vi "Decompose Map - Variant Mixed Value - Decomposes Successfully.vi"() -> ()   [LabVIEW 2019]
uses:
  <vilib>/addons/_JKI Toolkits/Caraya/classes/Assert/Assert Equal Value_Variant.vi
  Composition/Composition.lvlib
  <vilib>/addons/_JKI Toolkits/Caraya/classes/Test/Test.lvclass
  <vilib>/addons/_JKI Toolkits/Caraya/classes/Assert/Assert.lvclass
panel:
  out "error out":errorcluster
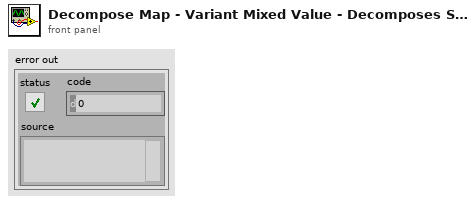
[diagram p1: front panel]
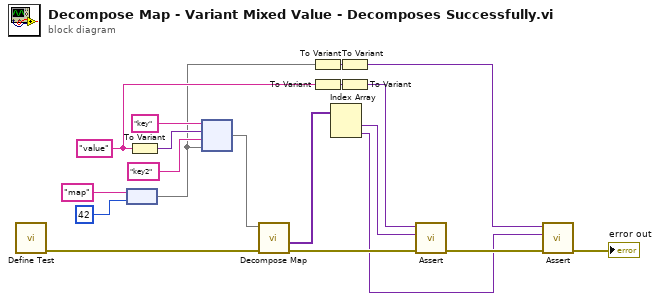
[diagram p0: block diagram]
diagram:
  w16 = "value" ("key")
  n1 = call <vilib>:"Define Test.vi"() -> ("error out"=w15:errorcluster)  [unwired: 10 in, 1 out]
  n2 = node("map" ("key"), 42 ("value")) -> (w2:map{string, i32})
  n3 = To Variant(anything=w16) -> (Variant=w14:variant)
  n4 = node("key" ("key"), w14, "key2" ("key"), w2) -> (w13:map{string, variant})
  n5 = call "Decompose Map.vi"("error in (no error)"=w15, "Variant Map"=w13) -> ("error out"=w18:errorcluster, "Values"=w12:variant[])  [unwired: 6 in, 2 out]
  n6 = To Variant(anything=w2) -> (Variant=w3:variant)
  n7 = To Variant(anything=w16) -> (Variant=w11:variant)
  n8 = Index Array(array=w12) -> (element #1=w17:variant, element #2=w4:variant)  [unwired: 2 in]
  n9 = To Variant(anything=w3) -> (Variant=w1:variant)
  n10 = To Variant(anything=w11) -> (Variant=w10:variant)
  n11 = call-poly <vilib>:"Assert.vi"("error in (no error)"=w18, "Y"=w17, "X"=w10) -> ("error out"=w6:errorcluster)  [unwired: 7 in, 1 out]
  n12 = call-poly <vilib>:"Assert.vi"("error in (no error)"=w6, "Y"=w4, "X"=w1) -> ("error out"=→"error out":errorcluster)  [unwired: 7 in, 1 out]
